vi "1c - Local variable.vi"() -> ()   [LabVIEW 2010]
panel:
  in  "stop":bool
  out "Chart 3":i32(graph)
  out "Chart 2":dbl(graph)
  out "Chart 1":dbl(graph)
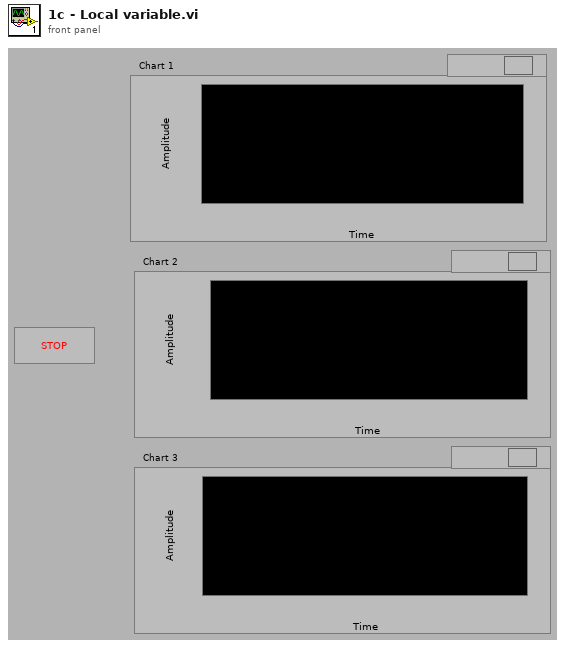
[diagram p1: front panel]
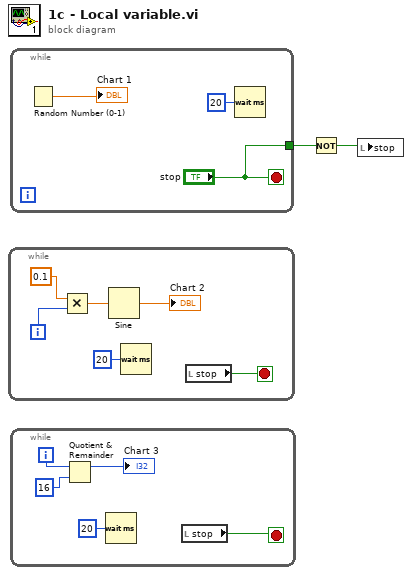
[diagram p0: block diagram]
diagram:
  n1 = while {
    i -> [w6]
    stop <- w3 stop-if-true
    n2 = Multiply(x=0.1, y=w6) -> (x*y=w5:dbl)
    n3 = Sine(x=w5) -> (sin(x)=→"Chart 2":dbl)
    n4 = Wait (ms)(milliseconds to wait=u32 20) -> ()  [unwired: 1 out]
    n5 = local read "stop"() -> (w3:bool)
  }
  n6 = while {
    tunnel: ["stop"] -> w2
    stop <- "stop" stop-if-true
    n7 = Random Number (0-1)() -> (number: 0 to 1=→"Chart 1":dbl)
    n8 = Wait (ms)(milliseconds to wait=u32 20) -> ()  [unwired: 1 out]
  }
  n9 = while {
    i -> [w15]
    stop <- w12 stop-if-true
    n10 = Quotient & Remainder(x=w15, y=16) -> (x-y*floor(x/y)=→"Chart 3":i32)  [unwired: 1 out]
    n11 = Wait (ms)(milliseconds to wait=u32 20) -> ()  [unwired: 1 out]
    n12 = local read "stop"() -> (w12:bool)
  }
  n13 = Not(x=w2) -> (.not. x?=w1:bool)
  n14 = local write "stop"(w1) -> ()
